vi "set_frequency.vi"(8 "error in (no error)":errorcluster, 10 "VISA resource name in":refnum<visa-resource-name>, 11 "Digital in":refnum<vi>) -> (0 "error out":errorcluster, 3 "VISA Refnum out":refnum<visa-resource-name>)   [LabVIEW 2021]
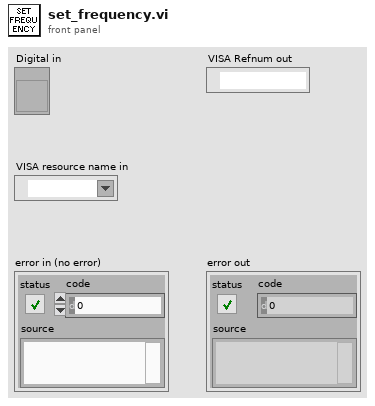
[diagram p1: front panel]
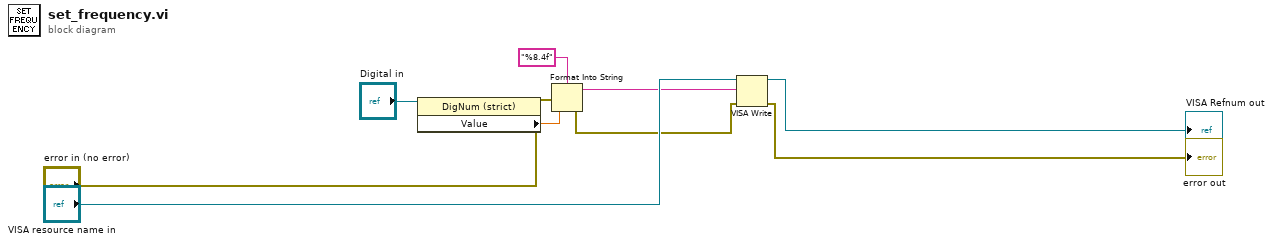
[diagram p0: block diagram]
diagram:
  n1 = property class="DigNum (strict)"(reference="Digital in") -> ("Value"=w2:dbl)  [unwired: 1 in, 2 out]
  n2 = Format Into String(format string="%8.4f", error in="error in (no error)", w2) -> (resulting string=w5:string, error out=w4:errorcluster)  [unwired: 1 in]
  n3 = VISA Write(VISA resource name="VISA resource name in", write buffer=w5, error in (no error)=w4) -> (VISA resource name out=→"VISA Refnum out":refnum<visa-resource-name>, error out=→"error out":errorcluster)  [unwired: 1 out]
